vi "Internal Data Exchange.vi"(8 "error in (no error)":errorcluster caption="Error In", 11 "Project":string) -> (0 "error out":errorcluster caption="Error Out", 3 "Write Data":map{string, string}(c390))   [LabVIEW 2020]
uses:
  0007 Controls/SY_Parameter.ctl
  Global/Data Global/Data Global Mode.ctl
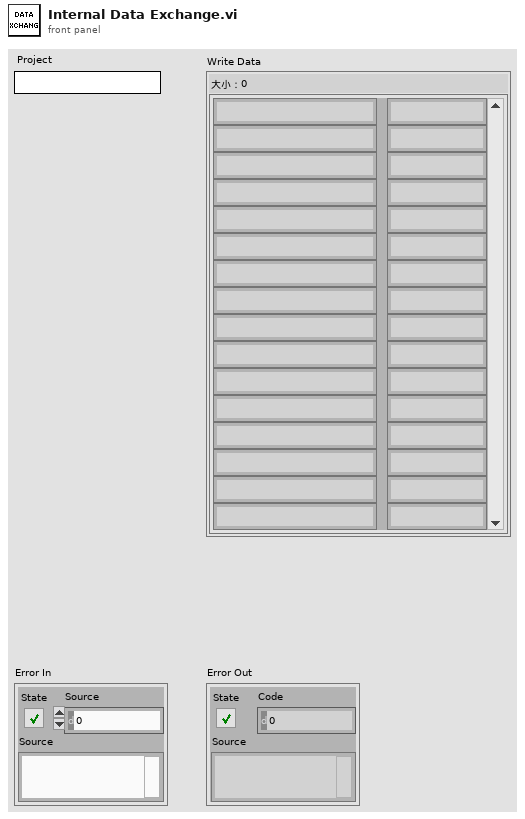
[diagram p1: front panel]
types:
  T1 = typedef "Data Global Mode.ctl" = enum16{"Init", "Read", "Write", "Write Data", "Load"}
  T2 = typedef "SY_Parameter.ctl" = cluster{"RH(%)":cluster{"DS":cluster{"阳极露点温度_DS":string, "阳极出口温度_DS":string, "阴极露点温度_DS":string, "阴极出口温度_DS":string, "阳极相对湿度_DS":string, "阴极相对湿度_DS":string, "阳极露点温度设置_DS":string, "阳极出口温度设置_DS":string, "阴极露点温度设置_DS":string, "阴极出口温度设置_DS":string}, "Value":cluster{"阳极露点温度_PV":sgl, "阳极出口温度_PV":sgl, "阴极露点温度_PV":sgl, "阴极出口温度_PV":sgl, "阳极相对湿度_SY":sgl, "阴极相对湿度_SY":sgl, "阳极露点温度设置_SV":sgl, "阳极出口温度设置_SV":sgl, "阴极露点温度设置_SV":sgl, "阴极出口温度设置_SV":sgl}}, "WEB":cluster{"DS":cluster{"自动模式(M0A1)_DS":string, "设备运行_DS":string, "工步号_DS":string, "运行模式_DS":string}, "Value":cluster{"自动模式(M0A1)_PV":bool, "设备运行_PV":bool, "工步号_PV":sgl, "运行模式_PV":bool}}, "ELD":cluster{"DS":cluster{"负载电压设置_DS":string, "负载电流设置_DS":string, "负载功率设置_DS":string, "负载模式设置_DS":string, "错误代码_DS":string, "负载电压_DS":string, "负载电流_DS":string, "负载功率_DS":string, "负载输出使能_DS":string, "负载连接_DS":string, "负载升压_DS":string, "负载升流_DS":string, "负载升功率_DS":string, "负载降压_DS":string, "负载降流_DS":string, "负载降功率_DS":string, "电流密度_DS":string, "功率密度_DS":string}, "Value":cluster{"负载电压设置_SV":sgl, "负载电流设置_SV":sgl, "负载功率设置_SV":sgl, "负载模式设置_SV":string, "错误代码_PV":string, "负载电压_PV":sgl, "负载电流_PV":sgl, "负载功率_PV":sgl, "负载输出使能_SV":bool, "负载连接_SY":bool, "负载升压_SV":sgl, "负载升流_SV":sgl, "负载升功率_SV":sgl, "负载降压_SV":sgl, "负载降流_SV":sgl, "负载降功率_SV":sgl, "电流密度_SV":sgl, "功率密度_SV":sgl}}, "SY":cluster{"DS":cluster{"总报警_DS":string, "WEB连接_DS":string, "计量比功能_DS":string, "PLC连接_DS":string, "H2计量比功能_DS":string, "Air计量比功能_DS":string, "PLC失联报警_DS":string}, "Value":cluster{"总报警_PV":bool, "WEB连接_PV":bool, "计量比功能_SV":bool, "PLC连接_SV":bool, "H2计量比功能_SV":bool, "Air计量比功能_SV":bool, "PLC失联报警_SV":bool}}, "PLC":cluster{"DS":cluster{"PLC急停_DS":string, "PLC连接_DS":string, "下位机心跳值_DS":string, "上位机心跳值_DS":string, "上位机报警等级字_DS":string, "负载可卸载_DS":string}, "Value":cluster{"PLC急停_PV":bool, "PLC连接_PV":bool, "下位机心跳值_PV":sgl, "上位机心跳值_SV":sgl, "上位机报警等级字_SV":sgl, "负载可卸载_SV":bool}}, "Bool Control":cluster{"DS":cluster{"维护模式_DS":string, "阳极氮气吹扫_DS":string, "阴极氮气吹扫_DS":string, "阳极脉冲使能_DS":string, "准备好使能_DS":string, "阳极干湿气切换_DS":string, "阴极干湿气切换_DS":string, "自动/手动模式_DS":string, "入口背压_DS":string, "手动卸载_DS":string, "软急停_DS":string, "负载连接_DS":string, "PLC故障复位_DS":string, "蜂鸣器屏蔽_DS":string}, "Value":cluster{"维护模式_SV":bool, "阳极氮气吹扫_SV":bool, "阴极氮气吹扫_SV":bool, "阳极脉冲使能_SV":bool, "准备好使能_SV":bool, "阳极干湿气切换_SV":bool, "阴极干湿气切换_SV":bool, "自动/手动模式_SV":bool, "入口背压_SV":bool, "手动卸载_SV":bool, "软急停_SV":bool, "负载连接_SV":bool, "PLC故障复位_SV":bool, "蜂鸣器屏蔽_SV":bool}}, "Stoich":cluster{"DS":cluster{"H2初始流量_DS":string, "Ait初始流量_DS":string, "H2侧系数_DS":string, "Air侧系数_DS":string, "H2计量比_DS":string, "Air计量比_DS":string, "时间间隔_DS":string, "H2计算气量_DS":string, "Air计算气量_DS":string, "H2流量_DS":string, "Air流量_DS":string}, "Value":cluster{"H2初始流量_SV":sgl, "Ait初始流量_SV":sgl, "H2侧系数_SV":sgl, "Air侧系数_SV":sgl, "H2计量比_SV":sgl, "Air计量比_SV":sgl, "时间间隔_SV":sgl, "H2计算气量_SV":sgl, "Air计算气量_SV":sgl, "H2流量_DS":sgl, "Air流量_DS":sgl}}, "PLC Need":cluster{"Name":string, "Identifier":string, "Source":string, "Value":string}[], "CVM":cluster{"DS":cluster{"活化面积_DS":string, "开路电压_DS":string, "单体总片数_DS":string, "单体显示片数_DS":string, "起始编号_DS":string, "最大值":string, "最大值编号_DS":string, "最小值_DS":string, "最小值编号_DS":string, "选区合计电压_DS":string, "平均值_DS":string, "离均差_DS":string}, "Value":cluster{"活化面积_SV":sgl, "开路电压_SV":sgl, "单体片数_SV":sgl, "单体显示片数_SV":sgl, "起始编号_SV":sgl, "最大值_SV":sgl, "最大值编号_SV":sgl, "最小值_SV":sgl, "最小值编号_SV":sgl, "选区合计电压_SV":sgl, "平均值_SV":sgl, "离均差_SV":sgl}}}
  T3 = cluster{"Write":map{string, string}, "Param Out":T2}
  T4 = cluster{"H2 Init Flow":sgl, "Air Init Flow":sgl, "H2 Coefficient":sgl, "Air Coefficient":sgl, "Stoic_H2":sgl, "Stoic_Air":sgl, "Piece":sgl, "Load Current":sgl}
  T5 = cluster{"Name":string, "Identifier":string, "Source":string, "Value":string}[]
  T6 = typedef "SDQ Data Type.ctl" = cluster{"CAN Length":string, "CAN Name":string, "CAN ID":string, "CAN Type":string, "Test Item":string, "Byte Order":string, "Instruction":string, "Control Type":string, "Group":string, "Offset":dbl, "Coefficient":dbl, "Write Enable":bool, "Lable Type":string, "Key?":string, "Set Value":string, "Upper":dbl, "Lower":dbl, "Unit":string, "Formula":string, "Test Item Type":string, "Length":i32, "Address":string, "Name":string, "Identifier":string, "Data Type":string, "Enumerate?":string, "Enumerate List":string, "Data":string, "Source":string}
  T7 = cluster{"阳极露点温度_PV":sgl, "阳极出口温度_PV":sgl, "阴极露点温度_PV":sgl, "阴极出口温度_PV":sgl, "阳极相对湿度_SY":sgl, "阴极相对湿度_SY":sgl, "阳极露点温度设置_SV":sgl, "阳极出口温度设置_SV":sgl, "阴极露点温度设置_SV":sgl, "阴极出口温度设置_SV":sgl}
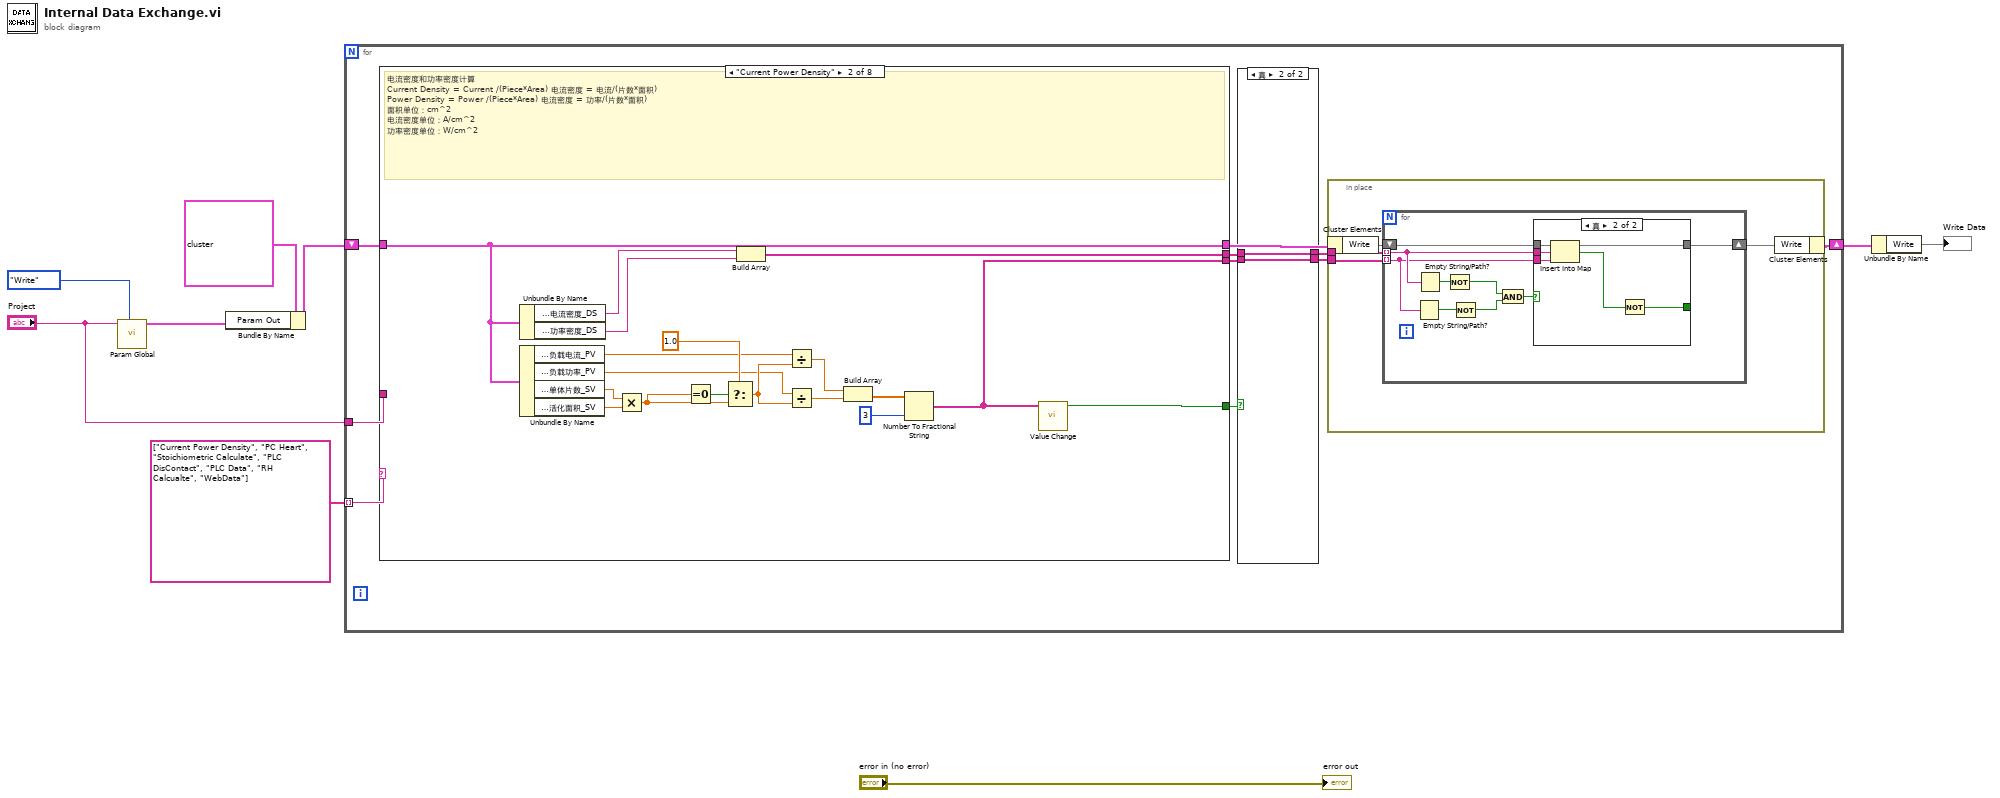
[diagram p0: block diagram]
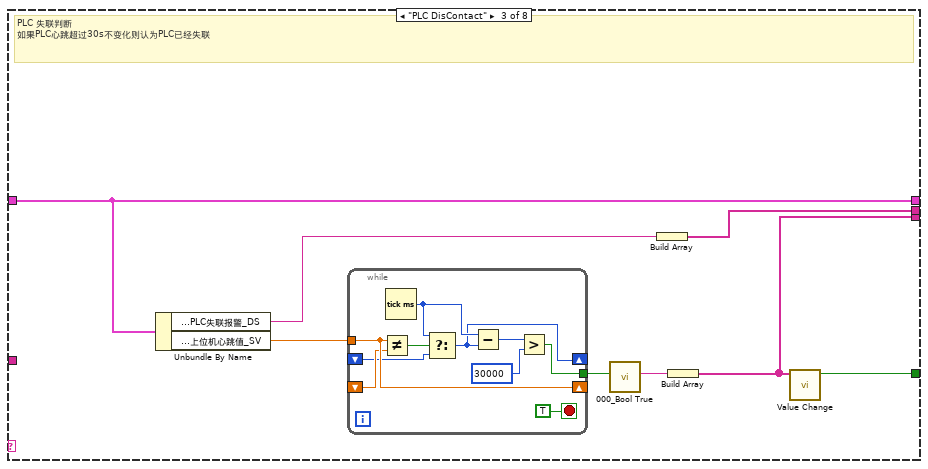
[diagram p5: hidden frame]
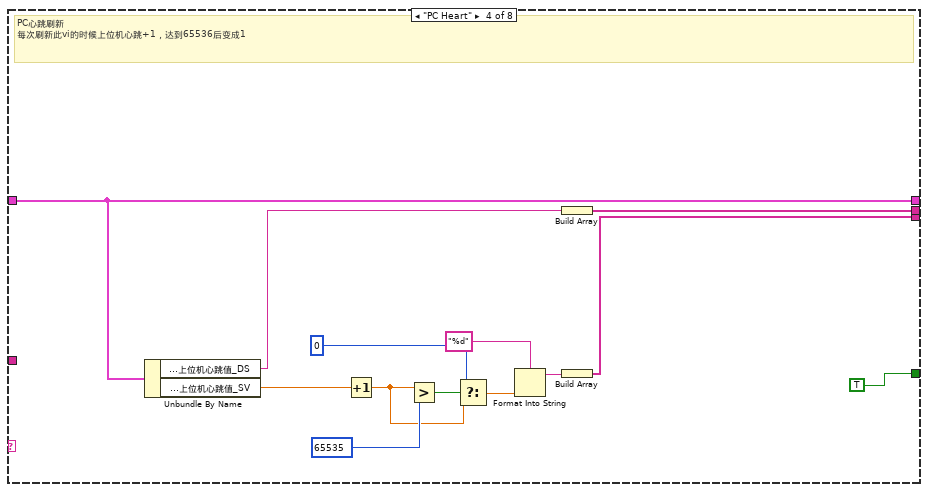
[diagram p6: hidden frame]
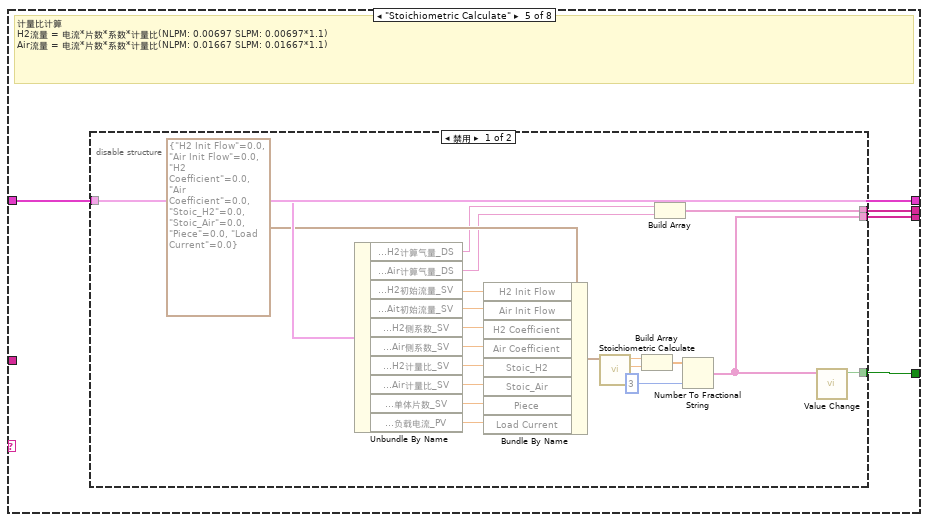
[diagram p7: hidden frame]
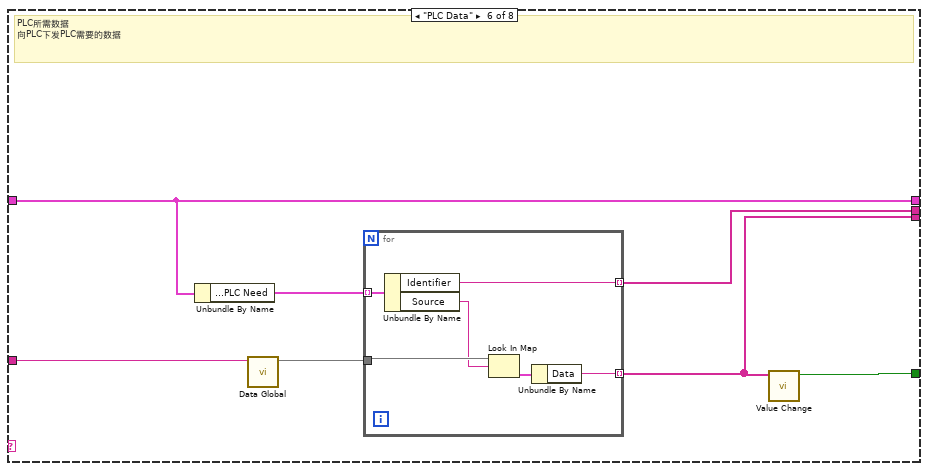
[diagram p9: hidden frame]
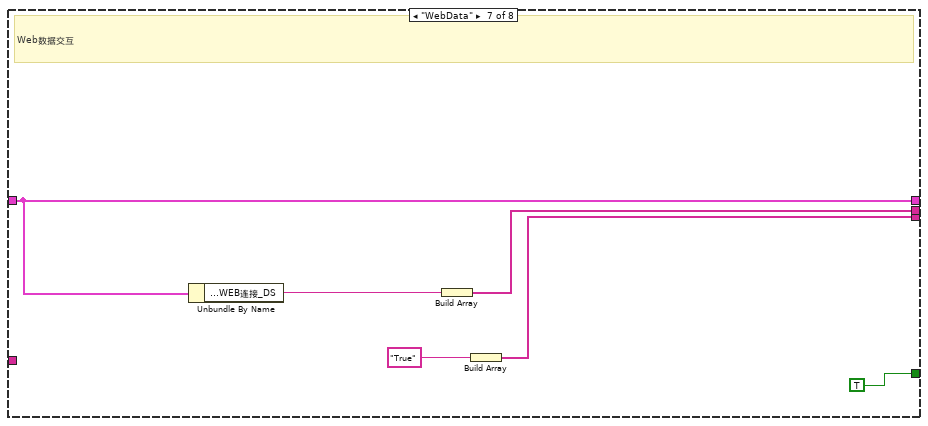
[diagram p10: hidden frame]
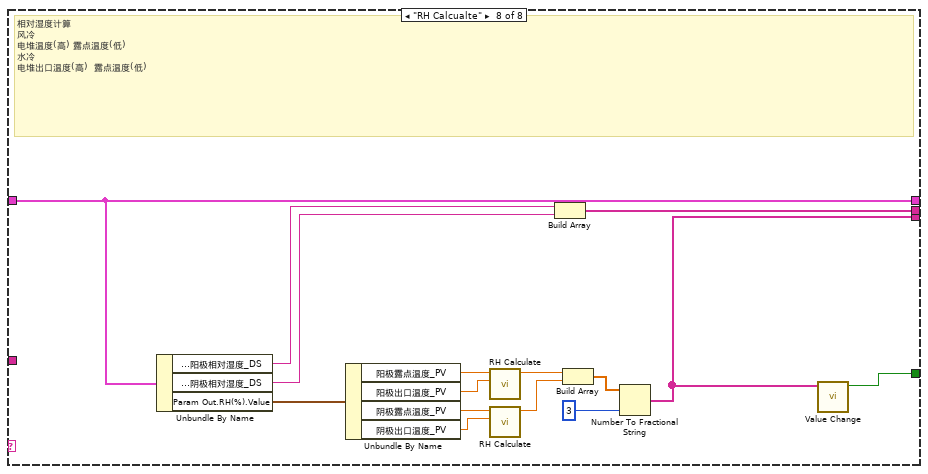
[diagram p11: hidden frame]
diagram:
  n1 = call "Param Global.vi"("Operate"=Data_Global_Mode."Write", "Project"="Project") -> ("Param Out"=w3:T2)  [unwired: 8 in, 1 out]
  n2 = Bundle By Name(cluster=T3 {"Write"={}, "Param Out"={"RH(%)"={"DS"={"阳极露点温度_DS"="TIRC101_PV", "阳极出口温度_DS"="TIR104_PV", "阴极露点温度_DS"="TIRC301_PV", "阴极出口温度_DS"="TIRC301_PV", "阳极相对湿度_DS"="SY_RH_An", "阴极相对湿度_DS"="SY_RH_Ca", "阳极露点温度设置_DS"="TIRC101_PV", "阳极出口温度设置_DS"="TIR104_PV", "阴极露点温度设置_DS"="TIRC301_PV", "阴极出口温度设置_DS"="TIRC301_PV"}, "Value"={"阳极露点温度_PV"=0.0, "阳极出口温度_PV"=0.0, "阴极露点温度_PV"=0.0, "阴极出口温度_PV"=0.0, "阳极相对湿度_SY"=0.0, "阴极相对湿度_SY"=0.0, "阳极露点温度设置_SV"=0.0, "阳极出口温度设置_SV"=0.0, "阴极露点温度设置_SV"=0.0, "阴极出口温度设置_SV"=0.0}}, "WEB"={"DS"={"自动模式(M0A1)_DS"="AUTO_MODE", "设备运行_DS"="DEVICE_STATE", "工步号_DS"="DEVICE_STATE", "运行模式_DS"="DEVICE_STATE"}, "Value"={"自动模式(M0A1)_PV"=FALSE, "设备运行_PV"=FALSE, "工步号_PV"=0.0, "运行模式_PV"=FALSE}}, "ELD"={"DS"={"负载电压设置_DS"="EL_V_SET", "负载电流设置_DS"="EL_A_SET", "负载功率设置_DS"="EL_P_SET", "负载模式设置_DS"="EL_MODE", "错误代码_DS"="EL_ERROR", "负载电压_DS"="EL_V", "负载电流_DS"="EL_A", "负载功率_DS"="EL_P", "负载输出使能_DS"="EL_INPUT", "负载连接_DS"="ELD", "负载升压_DS"="SY_Load_Rise_Volt", "负载升流_DS"="SY_Load_Rise_Curr", "负载升功率_DS"="SY_Load_Rise_Power", "负载降压_DS"="SY_Load_Drop_Volt", "负载降流_DS"="SY_Load_Drop_Curr", "负载降功率_DS"="SY_Load_Drop_Power", "电流密度_DS"="Density_A_SV", "功率密度_DS"="Density_P_SV"}, "Value"={"负载电压设置_SV"=0.0, "负载电流设置_SV"=0.0, "负载功率设置_SV"=0.0, "负载模式设置_SV"="", "错误代码_PV"="", "负载电压_PV"=0.0, "负载电流_PV"=0.0, "负载功率_PV"=0.0, "负载输出使能_SV"=FALSE, "负载连接_SY"=FALSE, "负载升压_SV"=0.0, "负载升流_SV"=0.0, "负载升功率_SV"=0.0, "负载降压_SV"=0.0, "负载降流_SV"=0.0, "负载降功率_SV"=0.0, "电流密度_SV"=0.0, "功率密度_SV"=0.0}}, "SY"={"DS"={"总报警_DS"="SY_Totol_Warning", "WEB连接_DS"="SY_Web_Con", "计量比功能_DS"="SY_Measurung_Ratio", "PLC连接_DS"="SY_Measurung_Ratio", "H2计量比功能_DS"="SY_Measurung_Ratio", "Air计量比功能_DS"="SY_Measurung_Ratio", "PLC失联报警_DS"="SY_Measurung_Ratio"}, "Value"={"总报警_PV"=FALSE, "WEB连接_PV"=FALSE, "计量比功能_SV"=FALSE, "PLC连接_SV"=FALSE, "H2计量比功能_SV"=FALSE, "Air计量比功能_SV"=FALSE, "PLC失联报警_SV"=FALSE}}, "PLC"={"DS"={"PLC急停_DS"="HMI_Estop_SV", "PLC连接_DS"="PLC", "下位机心跳值_DS"="PLC", "上位机心跳值_DS"="HMI_AlarmWord_SV", "上位机报警等级字_DS"="HMI_AlarmWord_SV", "负载可卸载_DS"="HMI_AlarmWord_SV"}, "Value"={"PLC急停_PV"=FALSE, "PLC连接_PV"=FALSE, "下位机心跳值_PV"=0.0, "上位机心跳值_SV"=0.0, "上位机报警等级字_SV"=0.0, "负载可卸载_SV"=FALSE}}, "Bool Control"={"DS"={"维护模式_DS"="WorkMode_SV", "阳极氮气吹扫_DS"="An_Purge_SV", "阴极氮气吹扫_DS"="Ca_Purge_SV", "阳极脉冲使能_DS"="An_Pulse_EN_SV", "准备好使能_DS"="DEVICE_READY", "阳极干湿气切换_DS"="An_GasMode_SV", "阴极干湿气切换_DS"="Ca_GasMode_SV", "自动/手动模式_DS"="AUTO_MODE", "入口背压_DS"="Stack_PreMode_SV", "手动卸载_DS"="HMI_Stack_OFF_SV", "软急停_DS"="HMI_Estop_SV", "负载连接_DS"="ELoad_EN_SV", "PLC故障复位_DS"="PLC_Alarm_Reset_SV", "蜂鸣器屏蔽_DS"="BuzzerShield_SV"}, "Value"={"维护模式_SV"=FALSE, "阳极氮气吹扫_SV"=FALSE, "阴极氮气吹扫_SV"=FALSE, "阳极脉冲使能_SV"=FALSE, "准备好使能_SV"=FALSE, "阳极干湿气切换_SV"=FALSE, "阴极干湿气切换_SV"=FALSE, "自动/手动模式_SV"=FALSE, "入口背压_SV"=FALSE, "手动卸载_SV"=FALSE, "软急停_SV"=FALSE, "负载连接_SV"=FALSE, "PLC故障复位_SV"=FALSE, "蜂鸣器屏蔽_SV"=FALSE}}, "Stoich"={"DS"={"H2初始流量_DS"="SY_Activation_Area", "Ait初始流量_DS"="SY_Pieces", "H2侧系数_DS"="SY_Activation_Area", "Air侧系数_DS"="SY_Pieces", "H2计量比_DS"="SY_Stoich_H2", "Air计量比_DS"="SY_Stoich_Air", "时间间隔_DS"="SY_Stoich_Interval", "H2计算气量_DS"="SY_Stoich_H2Flow", "Air计算气量_DS"="SY_Stoich_AirFlow", "H2流量_DS"="SY_Stoich_H2Flow", "Air流量_DS"="SY_Stoich_AirFlow"}, "Value"={"H2初始流量_SV"=0.0, "Ait初始流量_SV"=0.0, "H2侧系数_SV"=0.0, "Air侧系数_SV"=0.0, "H2计量比_SV"=0.0, "Air计量比_SV"=0.0, "时间间隔_SV"=0.0, "H2计算气量_SV"=0.0, "Air计算气量_SV"=0.0, "H2流量_DS"=0.0, "Air流量_DS"=0.0}}, "PLC Need"=[{"Name"="电堆电流_SV", "Identifier"="Stack_I_A_SV", "Source"="EL_A", "Value"=""}], "CVM"={"DS"={"活化面积_DS"="SY_Activation_Area", "开路电压_DS"="SY_OCV_Value", "单体总片数_DS"="SY_Pieces", "单体显示片数_DS"="SY_Pieces_Dis", "起始编号_DS"="SY_Starting_Number", "最大值"="SY_Activation_Area", "最大值编号_DS"="SY_OCV_Value", "最小值_DS"="SY_Pieces", "最小值编号_DS"="SY_Pieces_Dis", "选区合计电压_DS"="SY_Starting_Number", "平均值_DS"="SY_Pieces_Dis", "离均差_DS"="SY_Starting_Number"}, "Value"={"活化面积_SV"=0.0, "开路电压_SV"=0.0, "单体片数_SV"=0.0, "单体显示片数_SV"=0.0, "起始编号_SV"=0.0, "最大值_SV"=0.0, "最大值编号_SV"=0.0, "最小值_SV"=0.0, "最小值编号_SV"=0.0, "选区合计电压_SV"=0.0, "平均值_SV"=0.0, "离均差_SV"=0.0}}}}, "Param Out"=w3) -> (w7:T3)
  n3 = for {
    tunnel: string[] ["Current Power Density", "PC Heart", "Stoichiometric Calculate", "PLC DisContact", "PLC Data", "RH Calcualte", "WebData"] -> [w19] mode=indexing
    shift-right: [w16] -> w6
    shift-left: w7 -> [w18]
    tunnel: "Project" -> [w15]
    n4 = case shown="\"Current Power Density\"" w19 {
      tunnel: w18 -> [w42 w60 w68 w85 w94 w122 w134 w149]
      tunnel: [w42 w60 w68 w85 w94 w122 w134 w149] -> w17
      tunnel: [_ w57 w65 w80 w93 w119 w129 w147] -> w14
      tunnel: [_ w58 w67 w82 w95 w120 w132 w148] -> w13
      tunnel: w15 -> [_ _ _ _ _ w121 _ _]
      tunnel: [_ w59 w66 TRUE ("Change?") w92 w118 TRUE ("Change?") w146] -> w12
      frame "eee", Default {
      }
      frame "Current Power Density" {
        # "电流密度和功率密度计算\nCurrent Density = Current /(Piece*Area) 电流密度 = 电流/(片数*面积)\nPower Density = Power /(Piece*Area) 电流密度 = 功率/(片数*面积)\n面积单位：cm^2\n电流密度单位：A/cm^2\n功率密度单位：W/cm^2"
        n5 = Unbundle By Name(w60) -> ("Param Out.ELD.DS.电流密度_DS"=w50:string, "Param Out.ELD.DS.功率密度_DS"=w49:string)
        n6 = Unbundle By Name(w60) -> ("Param Out.ELD.Value.负载电流_PV"=w48:sgl, "Param Out.ELD.Value.负载功率_PV"=w47:sgl, "Param Out.CVM.Value.单体片数_SV"=w46:sgl, "Param Out.CVM.Value.活化面积_SV"=w45:sgl)
        n7 = Multiply(x=w46, y=w45) -> (x*y=w54:sgl)
        n8 = Equal To 0?(x=w54) -> (x = 0?=w56:bool)
        n9 = Select(t=1.0, s=w56, f=w54) -> (s? t:f=w53:dbl)
        n10 = Build Array(w50, w49) -> (w58:string[])
        n11 = Divide(x=w48, y=w53) -> (x/y=w52:dbl)
        n12 = Divide(x=w47, y=w53) -> (x/y=w51:dbl)
        n13 = Build Array(w52, w51) -> (w43:dbl[])
        n14 = Number To Fractional String(number=w43, precision (6)=i16 3 ("精度(6)")) -> (F-format string=w57:string[])  [unwired: 2 in]
        n15 = call "Value Change.vi"("New Data"=w57) -> ("Change?"=w59:bool)  [unwired: 10 in]
      }
      frame "PLC DisContact" {
        # "PLC 失联判断\n如果PLC心跳超过30s不变化则认为PLC已经失联"
        n16 = Unbundle By Name(w68) -> ("Param Out.SY.DS.PLC失联报警_DS"=w62:string, "Param Out.PLC.Value.上位机心跳值_SV"=w63:sgl)
        n17 = while {
          shift-right: [w77] -> _
          shift-left: _ -> [w76]
          tunnel: w63 -> [w77]
          shift-right: [w72] -> _
          shift-left: _ -> [w74]
          tunnel: [w69] -> w64
          stop <- TRUE stop-if-true
          n18 = Not Equal?(x=w77, y=w76) -> (x != y?=w75:bool)
          n19 = Tick Count (ms)() -> (millisecond timer value=w73:u32)
          n20 = Select(t=w73, s=w75, f=w74) -> (s? t:f=w72:u32)
          n21 = Subtract(x=w73, y=w72) -> (x-y=w71:u32)
          n22 = Greater?(x=w71, y=u32 30000) -> (0:w69:bool)
        }
        n23 = call "000_Bool True.vi"("Value"=w64) -> ("String Out"=w61:string)  [unwired: 8 in, 2 out]
        n24 = Build Array(w62) -> (w67:string[])
        n25 = Build Array(w61) -> (w65:string[])
        n26 = call "Value Change.vi"("New Data"=w65) -> ("Change?"=w66:bool)  [unwired: 10 in]
      }
      frame "PC Heart" {
        # "PC心跳刷新\n每次刷新此vi的时候上位机心跳+1，达到65536后变成1"
        n27 = Unbundle By Name(w85) -> ("Param Out.PLC.DS.上位机心跳值_DS"=w83:string, "Param Out.PLC.Value.上位机心跳值_SV"=w84:sgl)
        n28 = Increment(x=w84) -> (x+1=w87:sgl)
        n29 = Greater?(x=w87, y=65535) -> (0:w89:bool)
        n30 = Select(t=0, s=w89, f=w87) -> (s? t:f=w86:sgl)
        n31 = Format Into String(format string="%d" ("格式字符串"), w86) -> (resulting string=w81:string)  [unwired: 2 in, 1 out]
        n32 = Build Array(w83) -> (w82:string[])
        n33 = Build Array(w81) -> (w80:string[])
      }
      frame "Stoichiometric Calculate" {
        # "计量比计算\nH2流量 = 电流*片数*系数*计量比(NLPM: 0.00697 SLPM: 0.00697*1.1)\nAir流量 = 电流*片数*系数*计量比(NLPM: 0.01667 SLPM: 0.01667*1.1)"
        n34 = disable-structure shown="禁用" {
          disable-tunnel: [w111 _] -> w95
          disable-tunnel: w94 -> [w110 _]
          disable-tunnel: [w97 _] -> w93
          disable-tunnel: [w96 _] -> w92
          frame Disabled {
            n35 = Unbundle By Name(w110) -> ("Param Out.Stoich.DS.H2计算气量_DS"=w99:string, "Param Out.Stoich.DS.Air计算气量_DS"=w98:string, "Param Out.Stoich.Value.H2初始流量_SV"=w108:sgl, "Param Out.Stoich.Value.Ait初始流量_SV"=w101:sgl, "Param Out.Stoich.Value.H2侧系数_SV"=w102:sgl, "Param Out.Stoich.Value.Air侧系数_SV"=w103:sgl, "Param Out.Stoich.Value.H2计量比_SV"=w104:sgl, "Param Out.Stoich.Value.Air计量比_SV"=w105:sgl, "Param Out.CVM.Value.单体片数_SV"=w106:sgl, "Param Out.ELD.Value.负载电流_PV"=w107:sgl)
            n36 = Bundle By Name(cluster=T4 {"H2 Init Flow"=0.0, "Air Init Flow"=0.0, "H2 Coefficient"=0.0, "Air Coefficient"=0.0, "Stoic_H2"=0.0, "Stoic_Air"=0.0, "Piece"=0.0, "Load Current"=0.0}, "H2 Init Flow"=w108, "Air Init Flow"=w101, "H2 Coefficient"=w102, "Air Coefficient"=w103, "Stoic_H2"=w104, "Stoic_Air"=w105, "Piece"=w106, "Load Current"=w107) -> (w100:T4)
            n37 = call "Stoichiometric Calculate.vi"("Stoic Parameter"=w100) -> ("Air Flow"=w114:dbl, "H2 Flow"=w115:dbl)  [unwired: 9 in]
            n38 = Build Array(w115, w114) -> (w113:dbl[])
            n39 = Build Array(w99, w98) -> (w111:string[])
            n40 = Number To Fractional String(number=w113, precision (6)=i16 3 ("精度(6)")) -> (F-format string=w97:string[])  [unwired: 2 in]
            n41 = call "Value Change.vi"("New Data"=w97) -> ("Change?"=w96:bool)  [unwired: 10 in]
          }
          frame Enabled {
          }
        }
      }
      frame "PLC Data" {
        # "PLC所需数据\n向PLC下发PLC需要的数据"
        n42 = Unbundle By Name(w122) -> ("Param Out.PLC Need"=w117:T5)
        n43 = call "Data Global.vi"("Name"=w121) -> ("Data Out"=w116:map{string, T6})  [unwired: 7 in, 3 out]
        n44 = for {
          tunnel: w117 -> [w128] mode=indexing
          tunnel: w116 -> [w127]
          tunnel: [w124] -> w120 mode=indexing
          tunnel: [w123] -> w119 mode=indexing
          n45 = Unbundle By Name(w128) -> ("Identifier"=w124:string, "Source"=w126:string)
          n46 = Look In Map(map=w127, key=w126) -> (value=w125:T6)  [unwired: 1 in, 1 out]
          n47 = Unbundle By Name(w125) -> ("Data"=w123:string)
        }
        n48 = call "Value Change.vi"("New Data"=w119) -> ("Change?"=w118:bool)  [unwired: 10 in]
      }
      frame "WebData" {
        # "Web数据交互"
        n49 = Unbundle By Name(w134) -> ("Param Out.SY.DS.WEB连接_DS"=w133:string)
        n50 = Build Array(w133) -> (w132:string[])
        n51 = Build Array("True") -> (w129:string[])
      }
      frame "RH Calcualte" {
        # "相对湿度计算\n风冷\n电堆温度(高) 露点温度(低)\n水冷\n电堆出口温度(高)  露点温度(低)"
        n52 = Unbundle By Name(w149) -> ("Param Out.RH(%).DS.阳极相对湿度_DS"=w144:string, "Param Out.RH(%).DS.阴极相对湿度_DS"=w143:string, "Param Out.RH(%).Value"=w145:T7)
        n53 = Unbundle By Name(w145) -> ("阳极露点温度_PV"=w140:sgl, "阳极出口温度_PV"=w139:sgl, "阴极露点温度_PV"=w137:sgl, "阴极出口温度_PV"=w136:sgl)
        n54 = call "RH Calculate.vi"("T_饱和"=w139, "T_露点"=w140) -> ("RH(%)"=w138:sgl)  [unwired: 7 in, 2 out]
        n55 = call "RH Calculate.vi"("T_饱和"=w136, "T_露点"=w137) -> ("RH(%)"=w135:sgl)  [unwired: 7 in, 2 out]
        n56 = Build Array(w144, w143) -> (w148:string[])
        n57 = Build Array(w138, w135) -> (w141:sgl[])
        n58 = Number To Fractional String(number=w141, precision (6)=i16 3 ("精度(6)")) -> (F-format string=w147:string[])  [unwired: 2 in]
        n59 = call "Value Change.vi"("New Data"=w147) -> ("Change?"=w146:bool)  [unwired: 10 in]
      }
    }
    n60 = case shown="真" w12 {
      tunnel: w14 -> [_ w20]
      tunnel: w13 -> [_ w21]
      tunnel: [_ w21] -> w10
      tunnel: [_ w20] -> w11
      frame False {
      }
      frame True {
      }
    }
    n61 = in-place {
      in-place-border: w10 -> [w24]
      in-place-border: w11 -> [w22]
      n62 = in-place-cluster #1(w17) -> ("Write"=w25:map{string, string})
      n63 = for {
        shift-right: [w33] -> w23
        shift-left: w25 -> [w34]
        tunnel: w24 -> [w32] mode=indexing
        tunnel: w22 -> [w31] mode=indexing
        n64 = Empty String/Path?(string/path=w31) -> (empty?=w29:bool)
        n65 = Empty String/Path?(string/path=w32) -> (empty?=w30:bool)
        n66 = Not(x=w30) -> (.not. x?=w27:bool)
        n67 = Not(x=w29) -> (.not. x?=w26:bool)
        n68 = And(x=w27, y=w26) -> (x .and. y?=w28:bool)
        n69 = case shown="真" w28 {
          tunnel: w34 -> [w35 w41]
          tunnel: [w35 w40] -> w33
          tunnel: w32 -> [_ w39]
          tunnel: w31 -> [_ w38]
          tunnel: [_ w36] -> _
          frame False {
          }
          frame True {
            n70 = Insert Into Map(map in=w41, key=w39, value=w38) -> (map out=w40:map{string, string}, key already included?=w37:bool)  [unwired: 1 out]
            n71 = Not(x=w37) -> (.not. x?=w36:bool)
          }
        }
      }
      n72 = in-place-cluster #1("Write"=w23) -> (w16:T3)
    }
  }
  n73 = Unbundle By Name(w6) -> ("Write"=→"Write Data":map{string, string})
  "error out" <- "error in (no error)"
